vi "Production_count_SQL_data_fetch.vi"(5 "Current Shift":i32, 6 "error in (no error)":errorcluster, 7 "Cycle Data":T1={"CID"="", "Comm Stat"=FALSE, "Input"=[FALSE, FALSE, FALSE, FALSE, FALSE], "ip address's"="", "CYCLE COUNT"=0, "REJECTION COUNT"=0, "PRODUCT_CODE"=0, "ALARAM"=[FALSE, FALSE, FALSE, FALSE, FALSE, FALSE, FALSE, FALSE], "OUTPUT"=[FALSE, FALSE, FALSE, FALSE, FALSE], "PARTS PER HOUR"=0, "MR Retn Tmr"=0.0, "Holding Tmr"=0.0, "1st Pressure"=0.0, "2nd Pressure"=0.0}, 9 "Refnum in":T2) -> (0 "error out":errorcluster)   [LabVIEW 2017]
uses:
  <vilib>/addons/database/Connection.llb/Conn ObjectReference.ctl
  Control/Main_Data.ctl
  <vilib>/addons/database/Connection.llb/Conn Execute.vi
  <vilib>/addons/database/Recordset.llb/Rec Fetch Recordset Data (R).vi
  <vilib>/addons/database/Recordset.llb/Rec Destroy - Connection.vi
  <vilib>/addons/database/NI_Database_API.lvlib
panel:
  out "Date String":string
  out "date/time string":string
  out "PROD COUNT":i32
  out "Refnum out 2":T2
  out "PRODUCTION COUNT":i32
  out "TABLE NAME":string
  out "MAX BREAKDOWN ID":i32
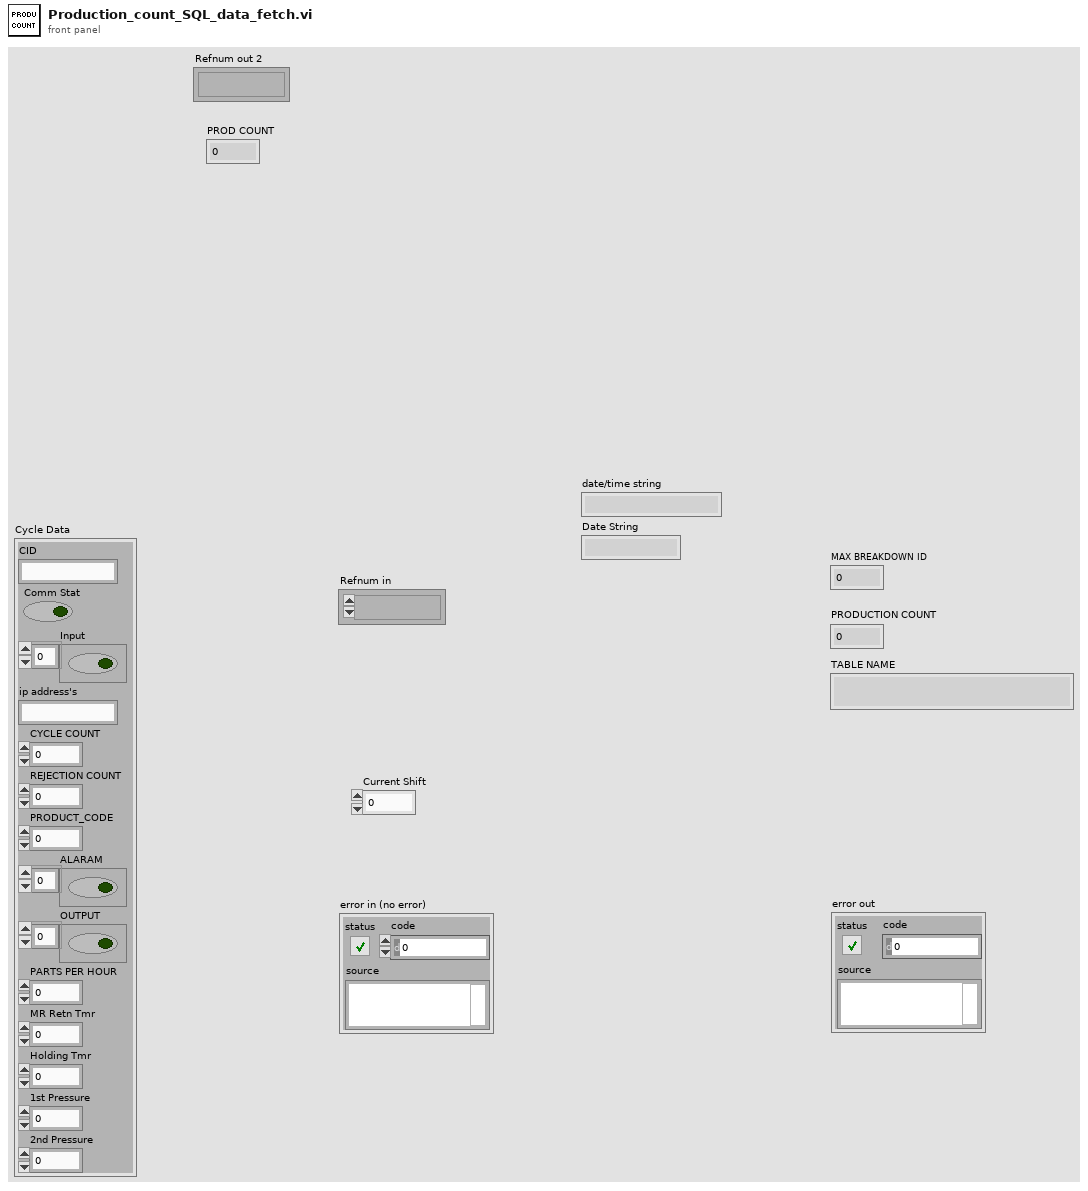
[diagram p1: front panel]
types:
  T1 = typedef "Main_Data.ctl" = cluster{"CID":string, "Comm Stat":bool, "Input":bool[], "ip address's":string, "CYCLE COUNT":u32, "REJECTION COUNT":u32, "PRODUCT_CODE":i16, "ALARAM":bool[], "OUTPUT":bool[], "PARTS PER HOUR":i16, "MR Retn Tmr":dbl, "Holding Tmr":dbl, "1st Pressure":dbl, "2nd Pressure":dbl}
  T2 = typedef "NI_Database_API.lvlib/Conn ObjectReference.ctl" = refnum<k1>
  T3 = typedef "NI_Database_API.lvlib/Rec ObjectReference.ctl" = refnum<k1>
  T4 = typedef "LVDateTimeRec.ctl" = cluster{"fractional second":dbl, "second":i32, "minute":i32, "hour":i32, "day of month":i32, "month":i32, "year":i32, "day of week":i32, "day of year":i32, "DST":i32}
  T5 = cluster{i32, "date/time string":string, "Current Shift":i32, "CID":string, "CYCLE COUNT":u32, "Date String":string, string, string}
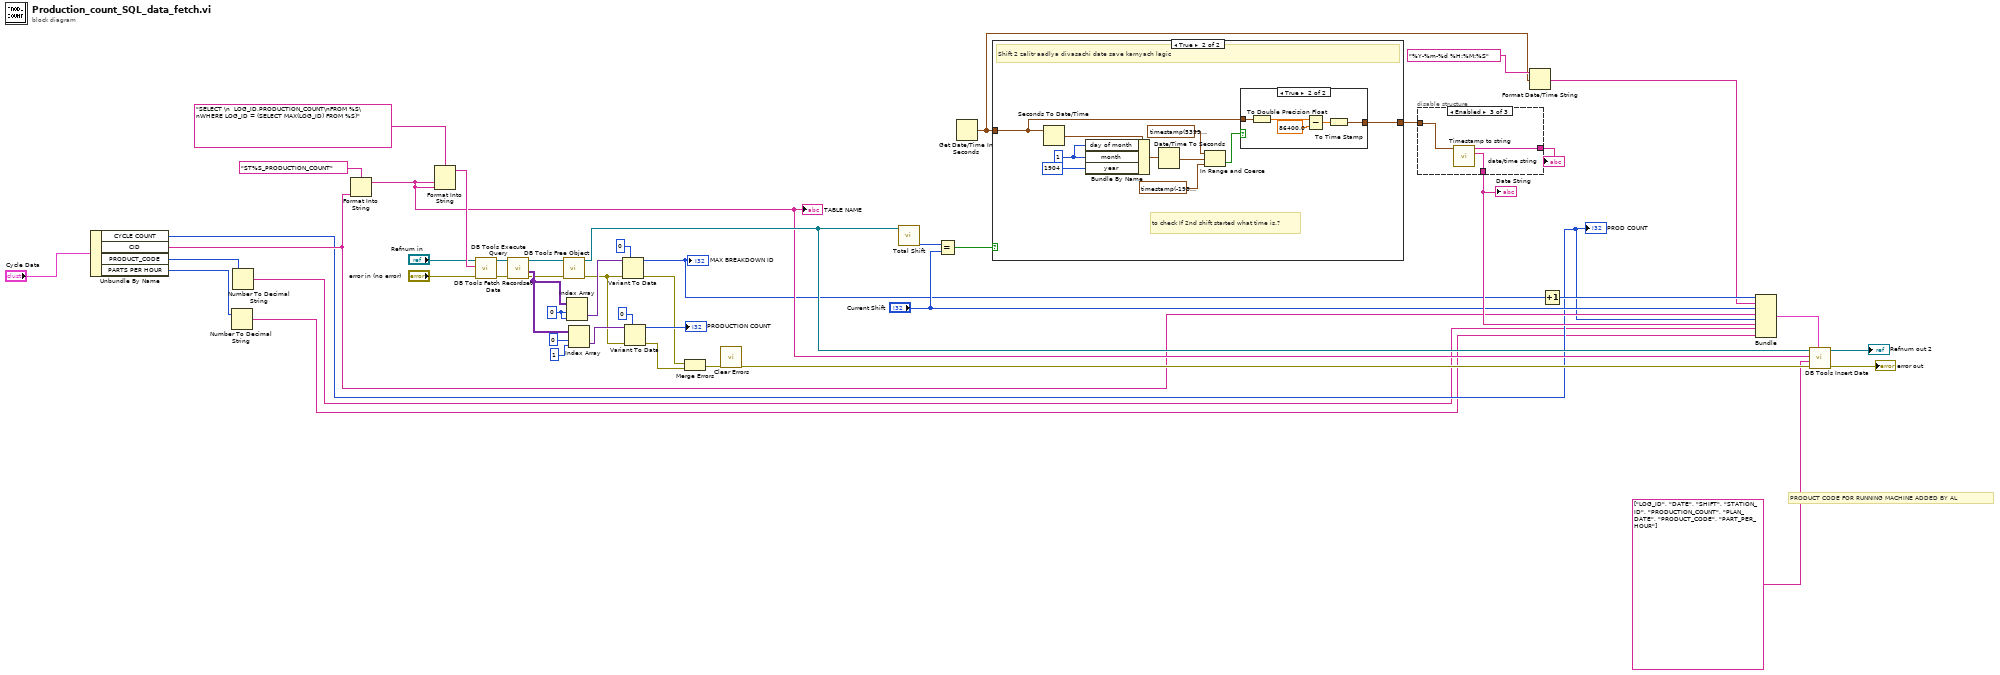
[diagram p0: block diagram]
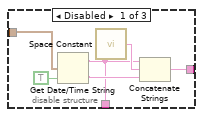
[diagram p2: hidden frame]
diagram:
  w42 = 0 ("index (row)")
  # "PRODUCT CODE FOR RUNNING MACHINE ADDED BY AL"
  n1 = Unbundle By Name("Cycle Data") -> ("CYCLE COUNT"=w3:u32, "CID"=w4:string, "PRODUCT_CODE"=w7:i16, "PARTS PER HOUR"=w6:i16)
  "PROD COUNT" <- w3
  n2 = Number To Decimal String(number=w6) -> (decimal integer string=w1:string)  [unwired: 1 in]
  n3 = Number To Decimal String(number=w7) -> (decimal integer string=w2:string)  [unwired: 1 in]
  n4 = Format Into String(format string="ST%S_PRODUCTION_COUNT" ("SQL query"), w4) -> (resulting string=w14:string)  [unwired: 2 in, 1 out]
  "TABLE NAME" <- w14
  n5 = Format Into String(format string="SELECT \n  LOG_ID,PRODUCTION_COUNT\nFROM %S\nWHERE LOG_ID = (SELECT MAX(LOG_ID) FROM %S)" ("SQL query"), w14, w14) -> (resulting string=w41:string)  [unwired: 2 in, 1 out]
  n6 = call-poly <vilib>:"DB Tools Execute Query.vi"("error in (no error)"="error in (no error)", "SQL query"=w41, "connection reference"="Refnum in") -> ("error out"=w45:errorcluster, "recordset reference"=w46:T3)  [unwired: 5 in]
  n7 = call-poly <vilib>:"DB Tools Fetch Recordset Data.vi"("error in (no error)"=w45, "recordset reference"=w46) -> ("error out"=w28:errorcluster, "recordset data"=w30:variant[][], "recordset reference out"=w47:T3)  [unwired: 3 in]
  n8 = call-poly <vilib>:"DB Tools Free Object.vi"("error in (no error)"=w28, "recordset reference"=w47) -> ("error out"=w25:errorcluster, "connection reference"=w16:T2)  [unwired: 8 in]
  n9 = Index Array(array=w30, index (row)=w42, index (col)=w42) -> (element=w43:variant)
  n10 = Index Array(array=w30, index (row)=0, index (col)=1) -> (element=w35:variant)
  n11 = Variant To Data(error in=w25, type=0, Variant=w43) -> (data=w12:i32, error out=w31:errorcluster)
  "MAX BREAKDOWN ID" <- w12
  n12 = Variant To Data(error in=w25, type=0, Variant=w35) -> (data=→"PRODUCTION COUNT":i32, error out=w32:errorcluster)
  n13 = Merge Errors(w31, w32) -> (w27:errorcluster)
  n14 = call <vilib>:"Clear Errors.vi"("error in (no error)"=w27) -> ("error out"=w26:errorcluster)  [unwired: 5 in, 1 out]
  n15 = call "Total Shift.vi"("connection reference"=w16) -> ("Total Shifts"=w18:i32)  [unwired: 9 in, 1 out]
  n16 = Equal?(x=w18, y="Current Shift") -> (x = y?=w19:bool)
  n17 = Get Date/Time In Seconds() -> (seconds since 1Jan1904=w8:timestamp)
  n18 = case shown="True" w19 {
    tunnel: w8 -> [w48 w49]
    tunnel: [w48 w50] -> w10
    frame False {
    }
    frame True {
      w55 = 1 ("day of month")
      # "to check If 2nd shift started what time is.?"
      # "Shift 2 zalitr aadlya divasachi date save karnyach lagic"
      n19 = Seconds To Date/Time(time stamp (now)=w49) -> (date time rec=w56:T4)  [unwired: 1 in]
      n20 = Bundle By Name(cluster=w56, "day of month"=w55, "month"=w55, "year"=1904) -> (w58:T4)
      n21 = Date/Time To Seconds(2:w58) -> (0:w54:timestamp)  [unwired: 1 in]
      n22 = In Range and Coerce(upper limit=timestamp(5399.999 s since 1904-01-01), x=w54, lower limit=timestamp(-19800 s since 1904-01-01)) -> (In Range?=w51:bool)  [unwired: 1 out]
      n23 = case shown="True" w51 {
        tunnel: [w59 w61] -> w50
        tunnel: w49 -> [w59 w60]
        frame False {
        }
        frame True {
          n24 = To Double Precision Float(number=w60) -> (double precision float=w64:dbl)
          n25 = Subtract(x=w64, y=86400.0) -> (x-y=w62:dbl)
          n26 = To Time Stamp(1:w62) -> (0:w61:timestamp)
        }
      }
    }
  }
  n27 = disable-structure shown="Enabled" {
    disable-tunnel: [w68 w71 w73] -> w21
    disable-tunnel: [w66 w71 w72] -> w20
    disable-tunnel: w10 -> [w65 w71 w74]
    frame Disabled {
      n28 = Get Date/Time String(seconds (now)=w65, want seconds? (F)=TRUE) -> (date string=w66:string, time string=w69:string)  [unwired: 1 in]
      n29 = call <vilib>:"Space Constant.vi"() -> ("String"=w70:string)
      n30 = Concatenate Strings(w66, w70, w69) -> (w68:string)
    }
    frame Disabled {
    }
    frame Enabled {
      n31 = call "Timestamp to string.vi"("time stamp"=w74) -> ("Date String"=w72:string, "date/time string"=w73:string)  [unwired: 8 in, 1 out]
    }
  }
  "date/time string" <- w21
  "Date String" <- w20
  n32 = Format Date/Time String(time format string (%c)="%Y-%m-%d %H:%M:%S", seconds (now)=w8) -> (date/time string=w9:string)  [unwired: 1 in]
  n33 = Increment(x=w12) -> (x+1=w22:i32)
  n34 = Bundle(w22, "date/time string"=w9, "Current Shift"="Current Shift", "CID"=w4, "CYCLE COUNT"=w3, "Date String"=w20, w2, w1) -> (w17:T5)  [unwired: 1 in]
  n35 = call <vilib>:"DB Tools Insert Data.vi"("data"=w17, "error in (no error)"=w26, "columns"=string[] ["LOG_ID", "DATE", "SHIFT", "STATION_ID", "PRODUCTION_COUNT", "PLAN_DATE", "PRODUCT_CODE", "PART_PER_HOUR"], "table"=w14, "connection reference"=w16) -> ("error out"=→"error out":errorcluster, "connection reference out"=→"Refnum out 2":T2)  [unwired: 5 in]
